vi "Init.vi"(8 "error in (no error)":errorcluster, 10 "Channel":i16=-10, 11 "AcquistionObject in":refnum<class "AcquistionObject.lvclass">) -> (0 "error out":errorcluster, 3 "AcquistionObject out":refnum<class "AcquistionObject.lvclass">)   [LabVIEW 2010, in "AcquistionObject.lvclass"]
uses:
  AcquistionObject.lvclass
  <vilib>/Utility/config.llb/Read Key (Path).vi
  <vilib>/Utility/config.llb/Read Key (String).vi
  <vilib>/addons/database/Connection.llb/DB Tools Open Connec (Path).vi
  <vilib>/Utility/config.llb/NI_LVConfig.lvlib
  <vilib>/addons/database/NI_Database_API.lvlib
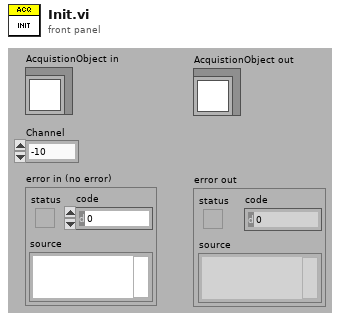
[diagram p1: front panel]
types:
  T1 = typedef "NI_LVConfig.lvlib/Config Data RefNum.ctl" = refnum<k1>
  T2 = typedef "NI_Database_API.lvlib/Conn ObjectReference.ctl" = refnum<k1>
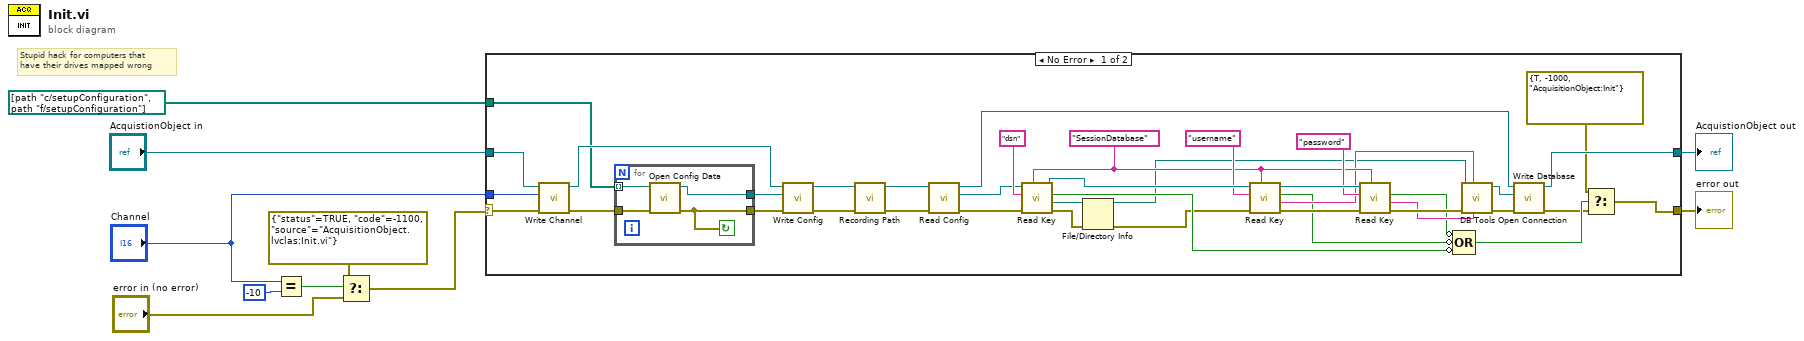
[diagram p0: block diagram]
diagram:
  # "Stupid hack for computers that \nhave their drives mapped wrong"
  n1 = Equal?(x="Channel", y=i16 -10 ("x")) -> (x = y?=w5:bool)
  n2 = Select(t=errorcluster {"status"=TRUE, "code"=-1100, "source"="AcquisitionObject.lvclas:Init.vi"}, s=w5, f="error in (no error)") -> (s? t:f=w3:errorcluster)
  n3 = case shown="No Error" w3 {
    selector: w3 -> [w12 w55]
    tunnel: [w27 w55] -> w10
    tunnel: [w43 w54] -> w8
    tunnel: "AcquistionObject in" -> [w20 w54]
    tunnel: path[] [path "c:/setupConfiguration", path "f:/setupConfiguration"] -> [w11 _]
    tunnel: "Channel" -> [w13 _]
    frame No Error {
      w36 = "SessionDatabase" ("section")
      n4 = call-dynamic "Write Channel.vi"("error in (no error)"=w12, "Channel"=w13, "AcquistionObject in"=w20) -> ("error out"=w19:errorcluster, "AcquistionObject out"=w15:refnum<class "AcquistionObject.lvclass">)  [unwired: 7 in]
      n5 = for {
        tunnel: w19 -> [w53]
        tunnel: [w52] -> w48
        tunnel: [w50] -> w47
        tunnel: w11 -> [w51] mode=indexing
        stop <- w50 continue-if-true
        n6 = call <vilib>:"Open Config Data.vi"("error in (no error)"=w53, "configuration file path"=w51) -> ("error out"=w50:errorcluster, "refnum"=w52:T1)  [unwired: 7 in, 1 out]
      }
      n7 = call-dynamic "Write Config.vi"("error in (no error)"=w47, "config data"=w48, "AcquistionObject in"=w15) -> ("error out"=w18:errorcluster, "AcquistionObject out"=w14:refnum<class "AcquistionObject.lvclass">)  [unwired: 7 in]
      n8 = call-dynamic "Recording Path.vi"("error in (no error)"=w18, "AcquistionObject in"=w14) -> ("error out"=w17:errorcluster, "AcquistionObject out"=w16:refnum<class "AcquistionObject.lvclass">)  [unwired: 7 in, 1 out]
      n9 = call-dynamic "Read Config.vi"("error in (no error)"=w17, "AcquistionObject in"=w16) -> ("error out"=w21:errorcluster, "config data"=w46:T1, "AcquistionObject out"=w22:refnum<class "AcquistionObject.lvclass">)  [unwired: 7 in]
      n10 = call-poly <vilib>:"Read Key.vi"("section"=w36, "error in (no error)"=w21, "key"="dsn", "refnum"=w46) -> ("error out"=w26:errorcluster, "value"=w24:path, "found?"=w31:bool, "refnum out"=w42:T1)  [unwired: 4 in]
      n11 = File/Directory Info(path=w24, error in=w26) -> (path out=w23:path, error out=w25:errorcluster)  [unwired: 5 out]
      n12 = call-poly <vilib>:"Read Key.vi"("section"=w36, "error in (no error)"=w25, "key"="username", "refnum"=w42) -> ("error out"=w40:errorcluster, "value"=w35:string, "found?"=w32:bool, "refnum out"=w39:T1)  [unwired: 4 in]
      n13 = call-poly <vilib>:"Read Key.vi"("section"=w36, "error in (no error)"=w40, "key"="password", "refnum"=w39) -> ("error out"=w37:errorcluster, "value"=w34:string, "found?"=w33:bool)  [unwired: 4 in, 1 out]
      n14 = Compound Arithmetic op=OR(invert w33, invert w32, invert w31) -> (w30:bool)
      n15 = call-poly <vilib>:"DB Tools Open Connection.vi"("password"=w34, "userID"=w35, "error in (no error)"=w37, "connection information"=w23) -> ("error out"=w45:errorcluster, "connection reference"=w44:T2)  [unwired: 4 in]
      n16 = call-dynamic "Write Database.vi"("error in (no error)"=w45, "reference"=w44, "AcquistionObject in"=w22) -> ("error out"=w29:errorcluster, "AcquistionObject out"=w43:refnum<class "AcquistionObject.lvclass">)  [unwired: 7 in]
      n17 = Select(t=errorcluster {"status"=TRUE, "code"=-1000, "source"="AcquisitionObject:Init"}, s=w30, f=w29) -> (s? t:f=w27:errorcluster)
    }
    frame Error {
    }
  }
  "error out" <- w10
  "AcquistionObject out" <- w8
